vi "Query Pulse Mode.vi"(6 "channel":i32=1 min=1 max=4, 8 "error in (no error)":errorcluster, 11 "VISA resource name":refnum<visa-resource-name>) -> (0 "error Out (no error)":errorcluster, 2 "Pulse Mode":u16(ring) items=["Single", "Double", "Triple", "Quadruple", "External Width"], 3 "VISA resource name out":refnum<visa-resource-name>)   [LabVIEW 2019, in "Pulse Rider PG-1000.lvlib"]
doc: "Query the pulse mode for the selected output channel. It sets how many pulses will be available for the selected output; if 'external width' is selected it means that the Trigger In signal is directly routed to the selected output.\n\nchannel: the output channel int from 1 to 4\nmode: an available mode : 'external width', 'quadruple', 'triple', 'double', 'single'"
uses:
  <instrlib>/Pulse Rider PG-1000/Pulse Rider PG-1000.lvlib
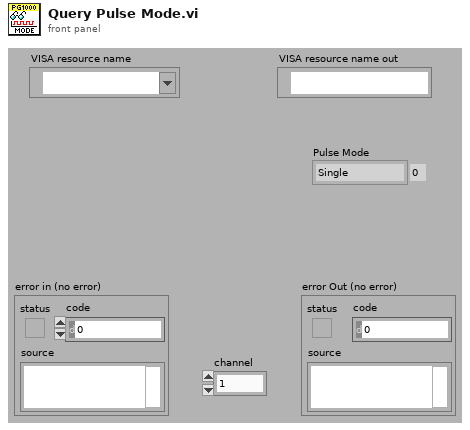
[diagram p1: front panel]
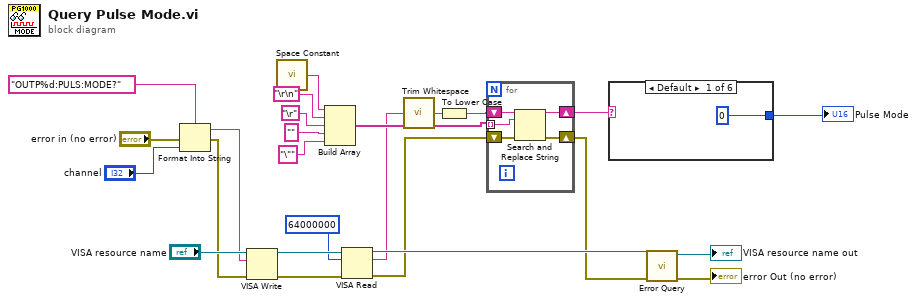
[diagram p0: block diagram]
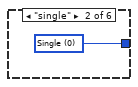
[diagram p2: hidden frame]
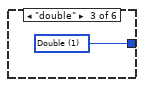
[diagram p3: hidden frame]
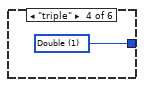
[diagram p4: hidden frame]
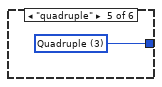
[diagram p5: hidden frame]
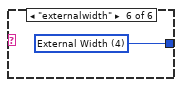
[diagram p6: hidden frame]
diagram:
  n1 = Format Into String(format string="OUTP%d:PULS:MODE?", error in="error in (no error)", "channel") -> (resulting string=w7:string, error out=w3:errorcluster)  [unwired: 1 in]
  n2 = VISA Write(VISA resource name="VISA resource name", write buffer=w7, error in (no error)=w3) -> (VISA resource name out=w22:refnum<visa-resource-name>, error out=w21:errorcluster)  [unwired: 1 out]
  n3 = call <vilib>:"Space Constant.vi"() -> ("String"=w18:string)
  n4 = Build Array(w18, "\r\n", "\r", "", "\"") -> (w13:string[])
  n5 = VISA Read(VISA resource name=w22, byte count=u32 64000000, error in (no error)=w21) -> (VISA resource name out=w19:refnum<visa-resource-name>, read buffer=w11:string, error out=w2:errorcluster)  [unwired: 1 out]
  n6 = call <vilib>:"Trim Whitespace.vi"("string"=w11) -> ("trimmed string"=w12:string)  [unwired: 1 in]
  n7 = To Lower Case(string=w12) -> (all lower case string=w10:string)
  n8 = for {
    tunnel: w13 -> [w28] mode=indexing
    shift-right: [w30] -> w6
    shift-left: w10 -> [w29]
    shift-right: [w26] -> w1
    shift-left: w2 -> [w27]
    n9 = Search and Replace String(input string=w29, search string=w28, error in=w27) -> (result string=w30:string, error out=w26:errorcluster)  [unwired: 5 in, 2 out]
  }
  n10 = case shown="Default" w6 {
    tunnel: [u16 0 ("Pulse Mode") w32 w33 w34 w35 w36] -> w5
    frame Default {
    }
    frame "single" {
      w32 = u16 0 items=["Single", "Double", "Triple", "Quadruple", "External Width"] ("Pulse Mode")
    }
    frame "double" {
      w33 = u16 1 items=["Single", "Double", "Triple", "Quadruple", "External Width"] ("Pulse Mode")
    }
    frame "triple" {
      w34 = u16 1 items=["Single", "Double", "Triple", "Quadruple", "External Width"] ("Pulse Mode")
    }
    frame "quadruple" {
      w35 = u16 3 items=["Single", "Double", "Triple", "Quadruple", "External Width"] ("Pulse Mode")
    }
    frame "externalwidth" {
      w36 = u16 4 items=["Single", "Double", "Triple", "Quadruple", "External Width"] ("Pulse Mode")
    }
  }
  "Pulse Mode" <- w5
  n11 = call <instrlib>:"Error Query.vi"("error in (no error)"=w1, "VISA resource name"=w19) -> ("error out"=→"error Out (no error)":errorcluster, "VISA resource name out"=→"VISA resource name out":refnum<visa-resource-name>)  [unwired: 6 in, 2 out]
